vi "device setup.vi"(7 "good pos":dbl[](array[numeric]) format="%.6f", 8 "error in (no error)":errorcluster caption="错误输入（无错误）") -> (0 "error out":errorcluster caption="错误输出", 2 "device index out":T1={"Position no."=1, "Rotaion no."=2, "piezo no."=3, "mg position"=0.0, "mg rotation"=0.0, "piezo position"=0.0, "pos axes"=[], "rot axes"=[], "piezo axes"=[]})   [LabVIEW 2017]
doc: "本VI用于在软件刚打开时进行仪器的通讯连接和校准，为之后控制仪器做准备。\n本VI无需输入，仅需运行时选择一次device ID (选1)，之后即自动完成平移电机，旋转电机，压电陶瓷的注册，校准，位移到中间的过程。\n本VI的仪器序列号仪器其他设置均作为常量设置在VI内，因为对于一套固定的仪器，这些参数是不修改的，为了避免仪器出错，不提供在主界面上修改的接口。\n本VI的基本执行顺序如下：\nVI开始执行，按参数注册平移电机1，选择电机，完成，注册旋转电机2，完成，注册压电陶瓷3，完成，报告平移电机位置，报告旋转电机位置，报告压电陶瓷位置，将电机编号NO. 和位置输入自定义控件中，作为输出值，供后续调用。\n本VI中还有一个禁用部分，是注销仪器注册的，在主程序中不启用，仅仅单个VI调试的时候启用。\n如果不注销，下次注册仪器就会占线出错。"
uses:
  device index.ctl
panel:
  out "error out 2":errorcluster
  in  "device index":T1={"Position no."=1, "Rotaion no."=2, "piezo no."=3, "mg position"=0.0, "mg rotation"=0.0, "piezo position"=0.0, "pos axes"=[], "rot axes"=[], "piezo axes"=[]}
  out "Identification 2":string
  out "SN out 2":string
  out "Device ID out 2":i32
  out "Identification":string
  out "SN out":string
  out "Device ID out":i32
  out "Position":dbl[](array[numeric]) format="%.6f"
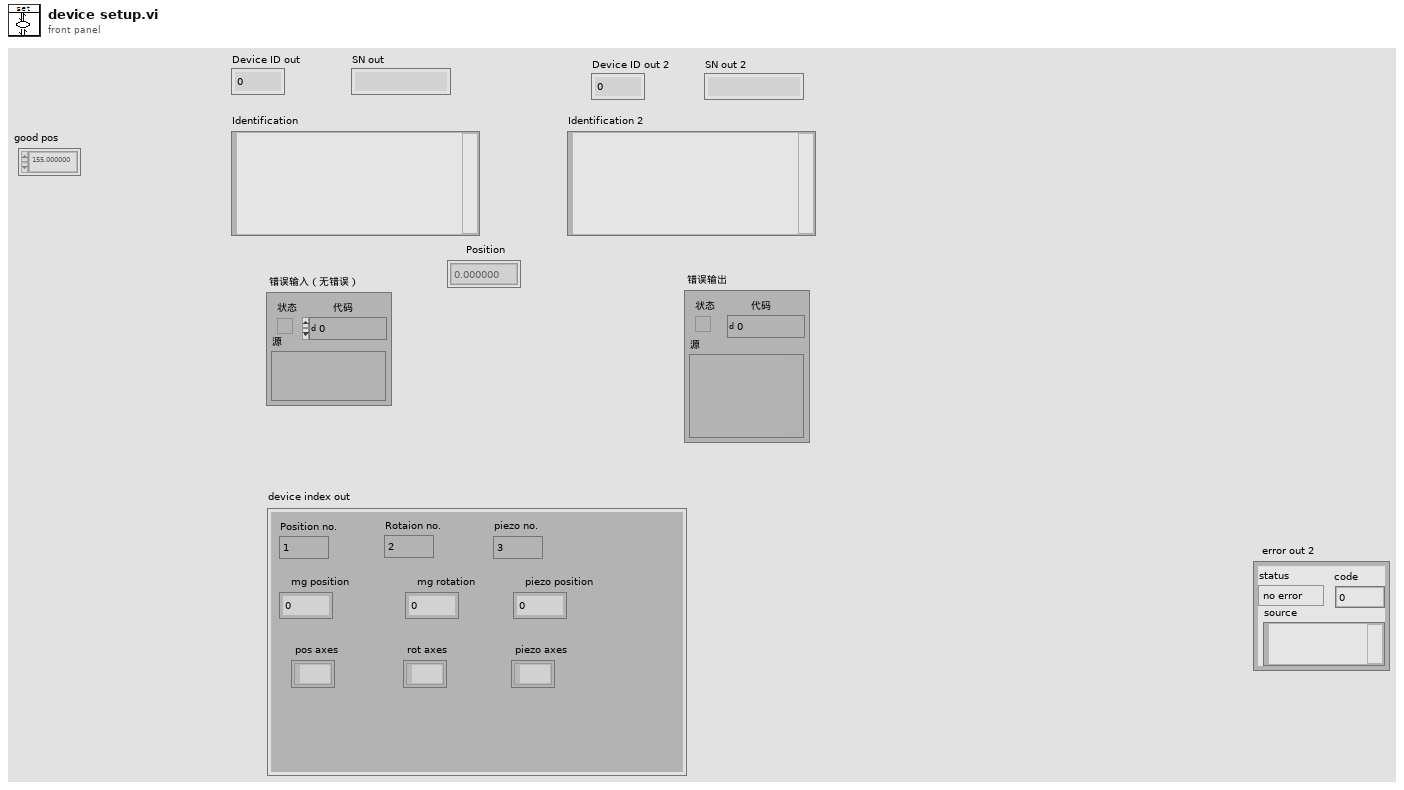
[diagram p1: front panel]
types:
  T1 = typedef "device index.ctl" = cluster{"Position no.":i32, "Rotaion no.":i32, "piezo no.":i32, "mg position":dbl, "mg rotation":dbl, "piezo position":dbl, "pos axes":string[], "rot axes":string[], "piezo axes":string[]}
  T2 = cluster{"RON Affected axes":string[], "Reference mode":bool[], "Check FRF?":bool}
  T3 = cluster{"Register DC":bool, "DaisyChain Search?":bool, "Device ID":i32}
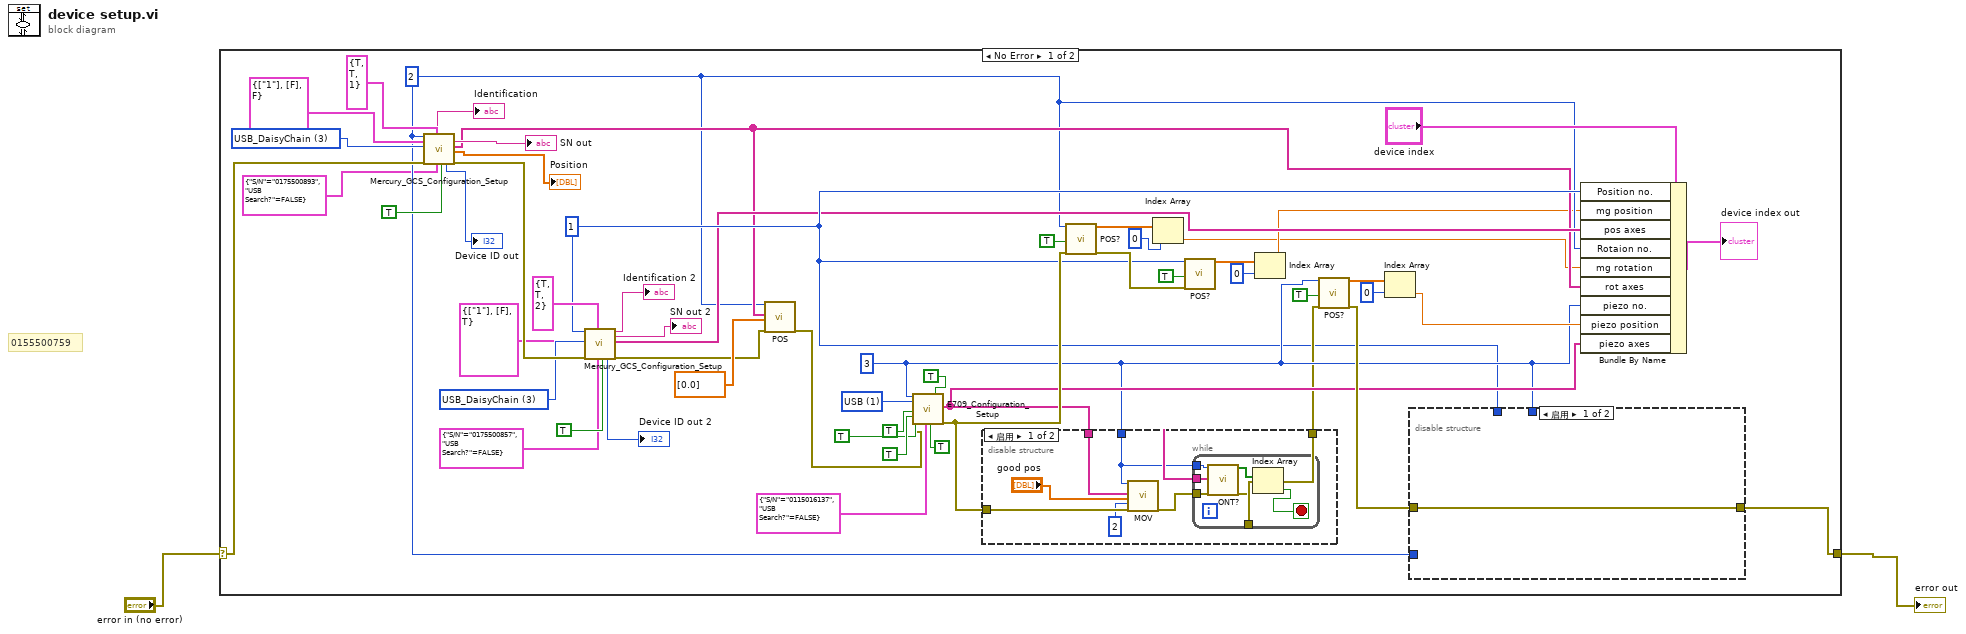
[diagram p0: block diagram]
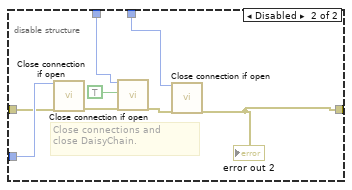
[diagram p3: hidden frame]
diagram:
  # "0155500759"
  n1 = case shown="No Error" "error in (no error)" {
    selector: "error in (no error)" -> [w55 w80]
    tunnel: [w30 w80] -> w1
    frame No Error {
      w36 = u16 1 items=["RS232", "USB"] ("Interface")
      w13 = 3 ("System no.")
      w46 = u16 3 items=["RS232", "RS232 DaisyChain", "USB", "USB_DaisyChain"] ("Interface")
      w56 = u16 3 items=["RS232", "RS232 DaisyChain", "USB", "USB_DaisyChain"] ("Interface")
      w10 = 1 ("System no.")
      w7 = 2 ("System no.")
      n2 = call "Mercury_GCS_Configuration_Setup.vi"("System no."=w7, "RON settings"=T2 {"RON Affected axes"=["1"], "Reference mode"=[FALSE], "Check FRF?"=FALSE}, "Interface"=w56, "error in"=w55, "DaisyChain settings"=T3 {"Register DC"=TRUE, "DaisyChain Search?"=TRUE, "Device ID"=1}, "USB settings"=cluster{"S/N":string, "USB Search?":bool} {"S/N"="0175500893", "USB Search?"=FALSE}, "Switch servo on?"=TRUE) -> ("Device ID out"=→"Device ID out":i32, "Identification"=→"Identification":string, "SN out"=→"SN out":string, "Conn. \nAxes"=w8:string[], "Position"=→"Position":dbl[], "error out"=w52:errorcluster)  [unwired: 6 in, 1 out]
      n3 = call "Mercury_GCS_Configuration_Setup.vi"("System no."=w10, "RON settings"=T2 {"RON Affected axes"=["1"], "Reference mode"=[FALSE], "Check FRF?"=TRUE}, "Interface"=w46, "error in"=w52, "DaisyChain settings"=T3 {"Register DC"=TRUE, "DaisyChain Search?"=TRUE, "Device ID"=2}, "USB settings"=cluster{"S/N":string, "USB Search?":bool} {"S/N"="0175500857", "USB Search?"=FALSE}, "Switch servo on?"=TRUE) -> ("Device ID out"=→"Device ID out 2":i32, "Identification"=→"Identification 2":string, "SN out"=→"SN out 2":string, "Conn. \nAxes"=w9:string[], "error out"=w17:errorcluster)  [unwired: 6 in, 2 out]
      n4 = call "POS.vi"("System no."=w7, "Axes to set"=w8, "Position values"=dbl[] [0.0], "error in"=w17) -> ("error out"=w16:errorcluster)  [unwired: 15 in]
      n5 = call "E709_Configuration_Setup.vi"("System no."=w13, "Interface"=w36, "Connected?"=TRUE, "Change servo status to ON?"=TRUE, "Perform autozero?"=TRUE, "error in"=w16, "USB settings"=cluster{"S/N":string, "USB Search?":bool} {"S/N"="0115016137", "USB Search?"=FALSE}, "Stop wave generator\noutput (if any)"=TRUE ("Stop wave generator\noutput (if any)"), "Move to middle?"=TRUE) -> ("Conn. \nAxis"=w14:string[], "error out"=w15:errorcluster)  [unwired: 5 in, 4 out]
      n6 = disable-structure shown="启用" {
        disable-tunnel: w15 -> [w63 w70]
        disable-tunnel: w14 -> [w59 _]
        disable-tunnel: w13 -> [w58 _]
        disable-tunnel: [w57 w70] -> w12
        frame Enabled {
          n7 = call "MOV.vi"("System no."=w58, "Axes to move"=w59, "Position values"="good pos", "No.of digits"=i16 2, "error in"=w63) -> ("error out"=w60:errorcluster)  [unwired: 14 in]
          n8 = while {
            tunnel: w60 -> [w69]
            tunnel: w59 -> [w68]
            tunnel: w58 -> [w67]
            tunnel: [w64] -> w57
            stop <- w65 stop-if-true
            n9 = call "ONT?.vi"("System no."=w67, "Axes to query"=w68, "error in"=w69) -> ("Axis on target?"=w66:bool[], "error out"=w64:errorcluster)  [unwired: 15 in]
            n10 = Index Array(array=w66) -> (element=w65:bool)  [unwired: 1 in]
          }
        }
        frame Disabled {
        }
      }
      n11 = call "POS?.vi"("System no."=w7, "All axes?"=TRUE, "error in"=w15) -> ("Position"=w28:dbl[], "error out"=w41:errorcluster)  [unwired: 15 in]
      n12 = Index Array(array=w28, index=0 ("索引")) -> (element=w5:dbl)
      n13 = call "POS?.vi"("System no."=w10, "All axes?"=TRUE, "error in"=w41) -> ("Position"=w25:dbl[])  [unwired: 15 in, 1 out]
      n14 = Index Array(array=w25, index=0 ("索引")) -> (element=w6:dbl)
      n15 = call "POS?.vi"("System no."=w13, "All axes?"=TRUE, "error in"=w12) -> ("Position"=w23:dbl[], "error out"=w31:errorcluster)  [unwired: 15 in]
      n16 = Index Array(array=w23, index=0 ("索引")) -> (element=w22:dbl)
      n17 = disable-structure shown="启用" {
        disable-tunnel: w7 -> [_ w76]
        disable-tunnel: w10 -> [_ w75]
        disable-tunnel: w13 -> [_ w74]
        disable-tunnel: w31 -> [w71 w73]
        disable-tunnel: [w71 w72] -> w30
        frame Enabled {
        }
        frame Disabled {
          # "Close connections and\nclose DaisyChain."
          n18 = call "Close connection if open.vi"("System no."=w76, "error in"=w73) -> ("error out"=w77:errorcluster)  [unwired: 16 in, 1 out]
          n19 = call "Close connection if open.vi"("System no."=w75, "Close DaisyChain"=TRUE, "error in"=w77) -> ("error out"=w79:errorcluster)  [unwired: 15 in, 1 out]
          n20 = call "Close connection if open.vi"("System no."=w74, "error in"=w79) -> ("error out"=w72:errorcluster)  [unwired: 16 in, 1 out]
          "error out 2" <- w72
        }
      }
      n21 = Bundle By Name(cluster="device index", "Position no."=w10, "mg position"=w6, "pos axes"=w9, "Rotaion no."=w7, "mg rotation"=w5, "rot axes"=w8, "piezo no."=w13, "piezo position"=w22, "piezo axes"=w14) -> (→"device index out":T1)
    }
    frame Error {
    }
  }
  "error out" <- w1
